vi "Last Element Read.vi"(4 "error in (no error)":errorcluster, 6 "Container State":T3, 7 "Display State In":T2 {"Time_data" format="%<%.3X>T"}) -> (0 "error out":errorcluster, 2 "Value":T1, 3 "Display State Out":T2 {"Time_data" format="%<%.3X>T"})   [LabVIEW 2013, in "Two Axis.xctl"]
uses:
  Two Axis.xctl
  <vilib>/_xctls/Container State.ctl
  Two Axis State.ctl
  <vilib>/_xctls/XControlSupport.lvlib
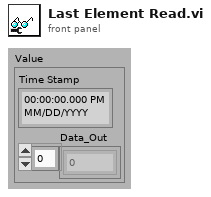
[diagram p1: front panel]
types:
  T1 = cluster{"Time Stamp":timestamp, "Data_Out":sgl[]}
  T2 = typedef "Two Axis.xctl/Two Axis State.ctl" = cluster{"History":i32, "Time_data":timestamp[], "Data_Out":sgl[][], "NumPlots":i32, "LegElem":i32, "Plot Details":cluster{"Name":string, "Line Width":u8, "Line Style":u8, "Color":u32}[], "Y-Axis Labels":string[], "Title":string, "data_only?":bool}
  T3 = typedef "XControlSupport.lvlib/Container State.ctl" = cluster{"Indicator?":bool, "Run Mode?":bool, " Refnum":refnum<vi>}
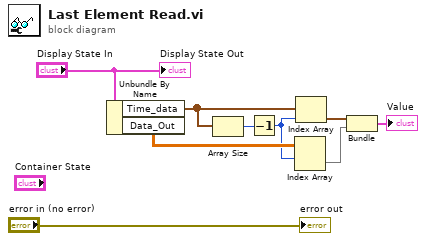
[diagram p0: block diagram]
diagram:
  n1 = Unbundle By Name("Display State In") -> ("Time_data"=w6:timestamp[], "Data_Out"=w5:sgl[][])
  n2 = Array Size(array=w6) -> (size(s)=w7:i32)
  n3 = Decrement(x=w7) -> (x-1=w4:i32)
  n4 = Index Array(array=w5, index (row)=w4) -> (element=w2:sgl[])  [unwired: 1 in]
  n5 = Index Array(array=w6, index=w4) -> (element=w3:timestamp)
  n6 = Bundle("Time Stamp"=w3, "Data_Out"=w2) -> (→"Value":T1)  [unwired: 1 in]
  "error out" <- "error in (no error)"
  "Display State Out" <- "Display State In"
